vi "Core.vi"(8 "error in (no error)":errorcluster, 11 "Serial in":refnum<class "Serial.lvclass">) -> (0 "error out":errorcluster, 3 "Serial out":refnum<class "Serial.lvclass">)   [LabVIEW 2021, in "Serial.lvclass"]
uses:
  Serial.lvclass
  D:/my_projects/projects/Algorithms/Labview/21/Master CR/Master CR.lvclass
  ctl/CR_Core_State.ctl
  Master CR.lvclass/Master CR.ctl
  Status/Run/Write Run.vi
  Status/write/Write write.vi
  Modbus_v121c/Data Model/Device Data Model.lvclass
  Serial.lvclass/Serial.ctl
  Master CR.lvclass
  D:/my_projects/projects/Algorithms/Labview/21/Master CR/Devices/Serial/Serial.lvclass
panel:
  out "MB_TCP_State":T1=enum."requests"
  in  "write enable":bool=TRUE
  in  "stop":bool
  out "stopped":bool
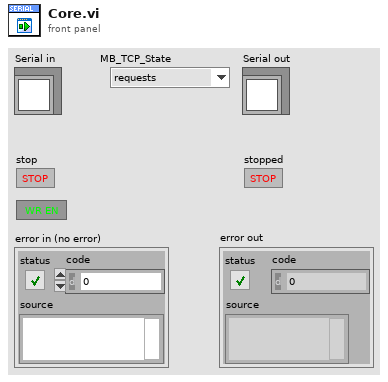
[diagram p1: front panel]
types:
  T1 = typedef "Master CR.lvclass/CR_Core_State.ctl" = enum8{"initialization", "redefine", "standby", "ping", "connect", "wait to reconnect", "wait to reset timeout", "configure", "requests", "close connection", "stop"}
  T2 = typedef "Master CR.lvclass/MB timeouts.ctl" = cluster{"reconn_timeout":i32, "N attempt max":i32, "t_reset_TTL":i32, "period":i32}
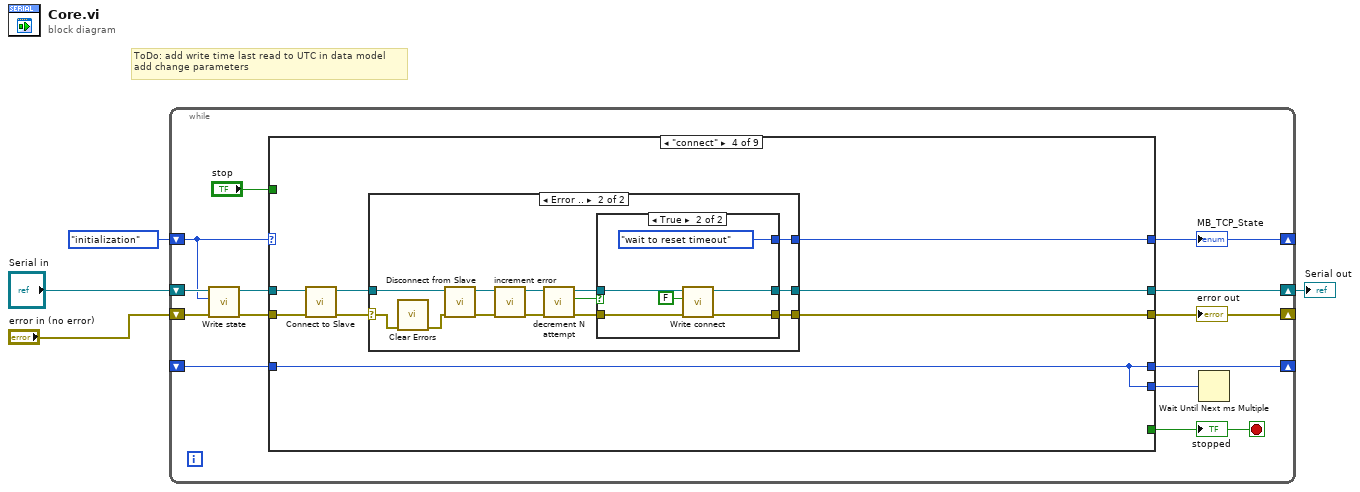
[diagram p0: block diagram]
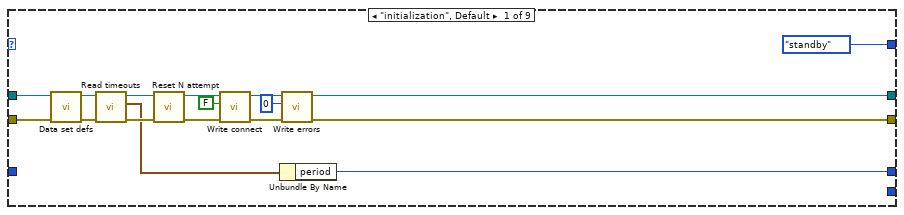
[diagram p2: hidden frame]
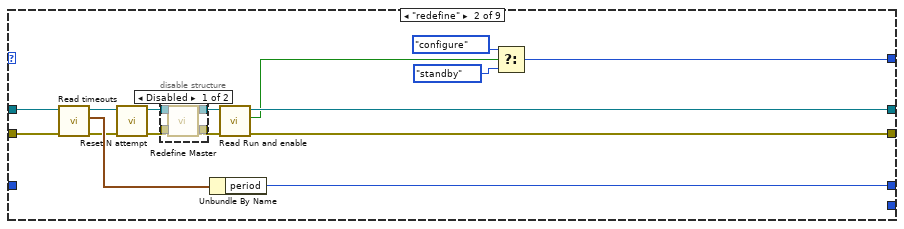
[diagram p3: hidden frame]
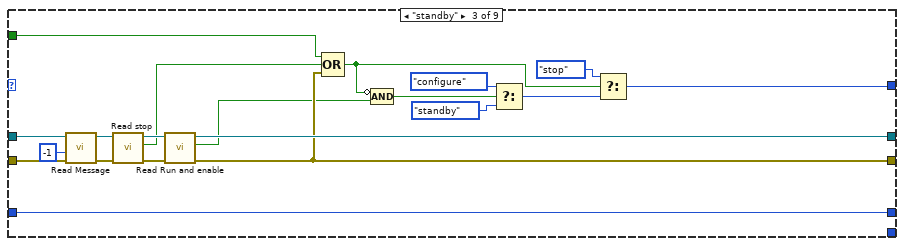
[diagram p5: hidden frame]
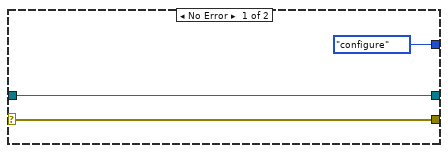
[diagram p6: hidden frame]
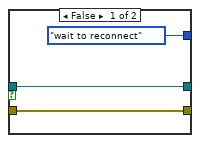
[diagram p7: hidden frame]
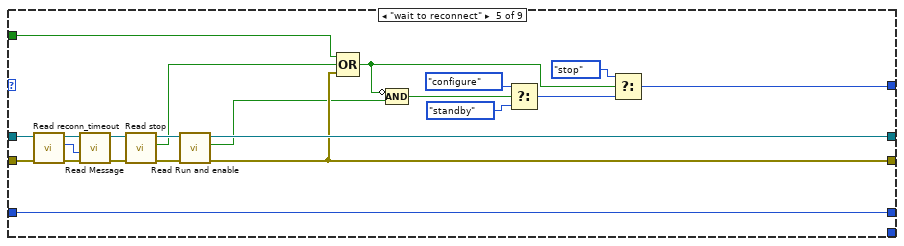
[diagram p8: hidden frame]
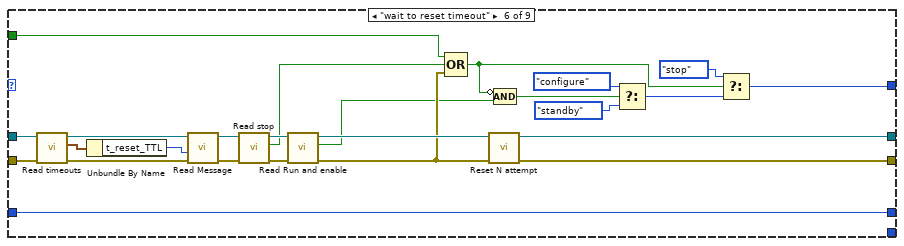
[diagram p9: hidden frame]
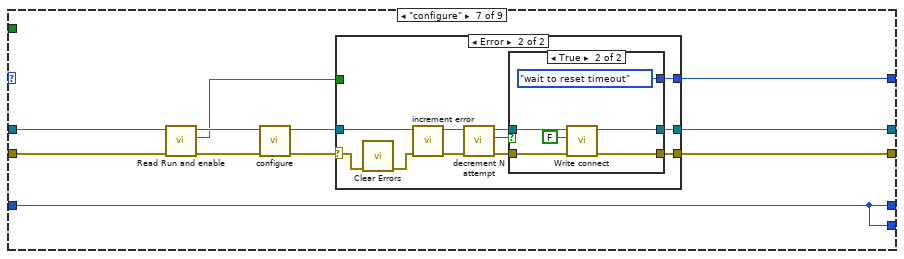
[diagram p10: hidden frame]
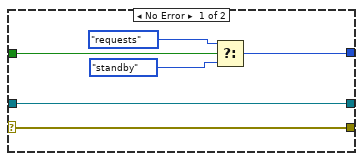
[diagram p11: hidden frame]
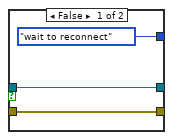
[diagram p12: hidden frame]
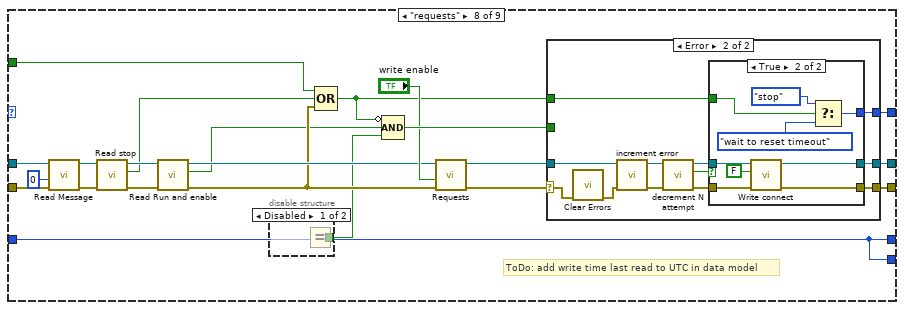
[diagram p13: hidden frame]
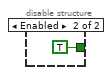
[diagram p14: hidden frame]
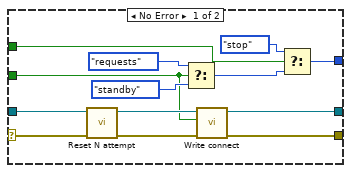
[diagram p15: hidden frame]
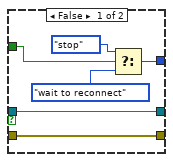
[diagram p16: hidden frame]
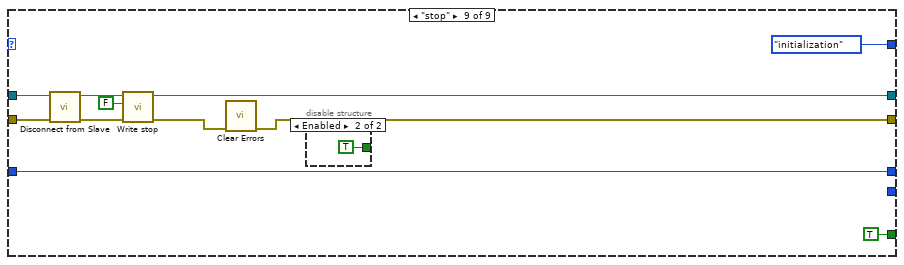
[diagram p17: hidden frame]
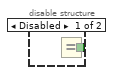
[diagram p18: hidden frame]
diagram:
  # "ToDo: add write time last read to UTC in data model\nadd change parameters"
  n1 = while {
    shift-right: [w10] -> w4
    shift-left: "Serial in" -> [w9]
    shift-right: [w11] -> _
    shift-left: "error in (no error)" -> [w7]
    shift-right: [w15] -> _
    shift-left: _ -> [w16]
    shift-right: [w12] -> _
    shift-left: CR_Core_State."initialization" ("state") -> [w5]
    stop <- w17 stop-if-true
    n2 = call "Write state.vi"("error in (no error)"=w7, "state"=w5, "Master CR in"=w9) -> ("error out"=w6:errorcluster, "Master CR out"=w8:refnum<class "Serial.lvclass">)  [unwired: 7 in]
    n3 = case shown="\"connect\"" w5 {
      tunnel: "stop" -> [_ _ w75 _ w119 w143 _ w205 _]
      tunnel: [_ _ _ _ _ _ _ _ TRUE] -> w17
      tunnel: w8 -> [w31 w47 w65 w80 w130 w155 w161 w207 w267]
      tunnel: [w20 w36 w67 w84 w117 w135 w167 w214 w260] -> w10
      tunnel: w6 -> [w32 w46 w64 w81 w129 w154 w160 w206 w266]
      tunnel: [CR_Core_State."standby" ("MB_TCP_State") w48 w68 w83 w118 w142 w166 w213 CR_Core_State."initialization" ("MB_TCP_State")] -> w12
      tunnel: [w18 w37 w66 w82 w116 w134 w165 w212 w265] -> w11
      tunnel: [w33 w44 w76 w77 w131 w156 w164 w210 w268] -> w15
      tunnel: w16 -> [_ _ w76 w77 w131 w156 w164 w210 w268]
      tunnel: [_ _ _ w77 _ _ w164 w210 _] -> w14
      frame "initialization", Default {
        n4 = call "Data set defs.vi"("error in (no error)"=w32, "Master CR in"=w31) -> ("error out"=w26:errorcluster, "Master CR out"=w29:refnum<class "Serial.lvclass">)  [unwired: 8 in]
        n5 = call "Read timeouts.vi"("error in (no error)"=w26, "Master CR in"=w29) -> ("error out"=w30:errorcluster, "MB timeouts"=w27:T2, "Master CR out"=w28:refnum<class "Serial.lvclass">)  [unwired: 7 in]
        n6 = call "Reset N attempt.vi"("error in (no error)"=w30, "Master CR in"=w28) -> ("error out"=w24:errorcluster, "Master CR out"=w25:refnum<class "Serial.lvclass">)  [unwired: 8 in]
        n7 = call "Write connect.vi"("error in (no error)"=w24, "connect"=FALSE, "Master CR in"=w25) -> ("error out"=w22:errorcluster, "Master CR out"=w21:refnum<class "Serial.lvclass">)  [unwired: 7 in]
        n8 = Unbundle By Name(w27) -> ("period"=w33:i32)
        n9 = call "Write errors.vi"("error in (no error)"=w22, "errors"=0, "Master CR in"=w21) -> ("error out"=w18:errorcluster, "Master CR out"=w20:refnum<class "Serial.lvclass">)  [unwired: 7 in]
      }
      frame "redefine" {
        n10 = call "Read timeouts.vi"("error in (no error)"=w46, "Master CR in"=w47) -> ("error out"=w43:errorcluster, "MB timeouts"=w45:T2, "Master CR out"=w42:refnum<class "Serial.lvclass">)  [unwired: 7 in]
        n11 = call "Reset N attempt.vi"("error in (no error)"=w43, "Master CR in"=w42) -> ("error out"=w40:errorcluster, "Master CR out"=w41:refnum<class "Serial.lvclass">)  [unwired: 8 in]
        n12 = disable-structure shown="Disabled" {
          disable-tunnel: w41 -> [w54 w56]
          disable-tunnel: w40 -> [w53 w55]
          disable-tunnel: [w52 w56] -> w39
          disable-tunnel: [w51 w55] -> w38
          frame Disabled {
            n13 = call "Redefine Master.vi"("error in (no error)"=w53, "Master CR in"=w54) -> ("error out"=w51:errorcluster, "Master CR out"=w52:refnum<class "Serial.lvclass">)  [unwired: 8 in]
          }
          frame Enabled {
          }
        }
        n14 = Unbundle By Name(w45) -> ("period"=w44:i32)
        n15 = call "Read Run and enable.vi"("error in (no error)"=w38, "Master CR in"=w39) -> ("error out"=w37:errorcluster, "Enable and Run"=w35:bool, "Master CR out"=w36:refnum<class "Serial.lvclass">)  [unwired: 7 in]
        n16 = Select(t=CR_Core_State."configure" ("MB_TCP_State"), s=w35, f=CR_Core_State."standby" ("MB_TCP_State")) -> (s? t:f=w48:T1)
      }
      frame "standby" {
        n17 = call "Read Message.vi"("error in (no error)"=w64, "timeout (0)"=-1, "Master CR in"=w65) -> ("error out"=w61:errorcluster, "Master CR out"=w62:refnum<class "Serial.lvclass">)  [unwired: 6 in, 1 out]
        n18 = call "Read stop.vi"("error in (no error)"=w61, "Master CR in"=w62) -> ("error out"=w60:errorcluster, "Stop"=w58:bool, "Master CR out"=w59:refnum<class "Serial.lvclass">)  [unwired: 7 in]
        n19 = call "Read Run and enable.vi"("error in (no error)"=w60, "Master CR in"=w59) -> ("error out"=w66:errorcluster, "Enable and Run"=w57:bool, "Master CR out"=w67:refnum<class "Serial.lvclass">)  [unwired: 7 in]
        n20 = Compound Arithmetic op=OR(w75, w58, w66) -> (w69:bool)
        n21 = Compound Arithmetic op=AND(invert w69, w57) -> (w70:bool)
        n22 = Select(t=CR_Core_State."configure" ("MB_TCP_State"), s=w70, f=CR_Core_State."standby" ("MB_TCP_State")) -> (s? t:f=w71:T1)
        n23 = Select(t=CR_Core_State."stop" ("MB_TCP_State"), s=w69, f=w71) -> (s? t:f=w68:T1)
      }
      frame "connect" {
        n24 = call-dynamic "Connect to Slave.vi"("error in (no error)"=w81, "network master in"=w80) -> ("error out"=w78:errorcluster, "network master out"=w79:refnum<class "Serial.lvclass">)  [unwired: 8 in]
        n25 = case shown="Error .." w78 {
          selector: w78 -> [w85 w92]
          tunnel: w79 -> [w86 w93]
          tunnel: [CR_Core_State."configure" ("MB_TCP_State") w98] -> w83
          tunnel: [w86 w97] -> w84
          tunnel: [w85 w96] -> w82
          frame No Error {
          }
          frame Error {
            n26 = call <vilib>:"Clear Errors.vi"("error in (no error)"=w92) -> ("error out"=w91:errorcluster)  [unwired: 5 in, 1 out]
            n27 = call-dynamic "Disconnect from Slave.vi"("error in (no error)"=w91, "network master in"=w93) -> ("error out"=w94:errorcluster, "network master out"=w95:refnum<class "Serial.lvclass">)  [unwired: 8 in]
            n28 = call "increment error.vi"("error in (no error)"=w94, "Master CR in"=w95) -> ("error out"=w90:errorcluster, "Master CR out"=w100:refnum<class "Serial.lvclass">)  [unwired: 7 in, 1 out]
            n29 = call "decrement N attempt.vi"("error in (no error)"=w90, "Master CR in"=w100) -> ("error out"=w88:errorcluster, "=0"=w99:bool, "Master CR out"=w89:refnum<class "Serial.lvclass">)  [unwired: 7 in]
            n30 = case shown="True" w99 {
              tunnel: [CR_Core_State."wait to reconnect" ("MB_TCP_State") CR_Core_State."wait to reset timeout" ("MB_TCP_State")] -> w98
              tunnel: w89 -> [w102 w105]
              tunnel: [w102 w108] -> w97
              tunnel: w88 -> [w101 w104]
              tunnel: [w101 w106] -> w96
              frame False {
              }
              frame True {
                n31 = call "Write connect.vi"("error in (no error)"=w104, "connect"=FALSE, "Master CR in"=w105) -> ("error out"=w106:errorcluster, "Master CR out"=w108:refnum<class "Serial.lvclass">)  [unwired: 7 in]
              }
            }
          }
        }
      }
      frame "wait to reconnect" {
        n32 = call "Read reconn_timeout.vi"("error in (no error)"=w129, "Master CR in"=w130) -> ("error out"=w120:errorcluster, "reconn_timeout"=w121:i32, "Master CR out"=w122:refnum<class "Serial.lvclass">)  [unwired: 7 in]
        n33 = call "Read Message.vi"("error in (no error)"=w120, "timeout (0)"=w121, "Master CR in"=w122) -> ("error out"=w114:errorcluster, "Master CR out"=w115:refnum<class "Serial.lvclass">)  [unwired: 6 in, 1 out]
        n34 = call "Read stop.vi"("error in (no error)"=w114, "Master CR in"=w115) -> ("error out"=w113:errorcluster, "Stop"=w111:bool, "Master CR out"=w112:refnum<class "Serial.lvclass">)  [unwired: 7 in]
        n35 = call "Read Run and enable.vi"("error in (no error)"=w113, "Master CR in"=w112) -> ("error out"=w116:errorcluster, "Enable and Run"=w110:bool, "Master CR out"=w117:refnum<class "Serial.lvclass">)  [unwired: 7 in]
        n36 = Compound Arithmetic op=OR(w119, w111, w116) -> (w123:bool)
        n37 = Compound Arithmetic op=AND(invert w123, w110) -> (w124:bool)
        n38 = Select(t=CR_Core_State."configure" ("MB_TCP_State"), s=w124, f=CR_Core_State."standby" ("MB_TCP_State")) -> (s? t:f=w125:T1)
        n39 = Select(t=CR_Core_State."stop" ("MB_TCP_State"), s=w123, f=w125) -> (s? t:f=w118:T1)
      }
      frame "wait to reset timeout" {
        n40 = call "Read timeouts.vi"("error in (no error)"=w154, "Master CR in"=w155) -> ("error out"=w146:errorcluster, "MB timeouts"=w153:T2, "Master CR out"=w145:refnum<class "Serial.lvclass">)  [unwired: 7 in]
        n41 = Unbundle By Name(w153) -> ("t_reset_TTL"=w144:i32)
        n42 = call "Read Message.vi"("error in (no error)"=w146, "timeout (0)"=w144, "Master CR in"=w145) -> ("error out"=w139:errorcluster, "Master CR out"=w141:refnum<class "Serial.lvclass">)  [unwired: 6 in, 1 out]
        n43 = call "Read stop.vi"("error in (no error)"=w139, "Master CR in"=w141) -> ("error out"=w138:errorcluster, "Stop"=w137:bool, "Master CR out"=w140:refnum<class "Serial.lvclass">)  [unwired: 7 in]
        n44 = call "Read Run and enable.vi"("error in (no error)"=w138, "Master CR in"=w140) -> ("error out"=w133:errorcluster, "Enable and Run"=w132:bool, "Master CR out"=w136:refnum<class "Serial.lvclass">)  [unwired: 7 in]
        n45 = Compound Arithmetic op=OR(w143, w137, w133) -> (w147:bool)
        n46 = call "Reset N attempt.vi"("error in (no error)"=w133, "Master CR in"=w136) -> ("error out"=w134:errorcluster, "Master CR out"=w135:refnum<class "Serial.lvclass">)  [unwired: 8 in]
        n47 = Compound Arithmetic op=AND(invert w147, w132) -> (w148:bool)
        n48 = Select(t=CR_Core_State."configure" ("MB_TCP_State"), s=w148, f=CR_Core_State."standby" ("MB_TCP_State")) -> (s? t:f=w149:T1)
        n49 = Select(t=CR_Core_State."stop" ("MB_TCP_State"), s=w147, f=w149) -> (s? t:f=w142:T1)
      }
      frame "configure" {
        n50 = call "Read Run and enable.vi"("error in (no error)"=w160, "Master CR in"=w161) -> ("error out"=w158:errorcluster, "Enable and Run"=w157:bool, "Master CR out"=w159:refnum<class "Serial.lvclass">)  [unwired: 7 in]
        n51 = call-dynamic "configure.vi"("error in (no error)"=w158, "Master CR in"=w159) -> ("error out"=w162:errorcluster, "Master CR out"=w163:refnum<class "Serial.lvclass">)  [unwired: 8 in]
        n52 = case shown="Error" w162 {
          selector: w162 -> [w169 w184]
          tunnel: [w173 w174] -> w166
          tunnel: [w169 w177] -> w165
          tunnel: w163 -> [w170 w176]
          tunnel: [w170 w178] -> w167
          tunnel: w157 -> [w168 _]
          frame No Error {
            n53 = Select(t=CR_Core_State."requests" ("MB_TCP_State"), s=w168, f=CR_Core_State."standby" ("MB_TCP_State")) -> (s? t:f=w173:T1)
          }
          frame Error {
            n54 = call <vilib>:"Clear Errors.vi"("error in (no error)"=w184) -> ("error out"=w175:errorcluster)  [unwired: 5 in, 1 out]
            n55 = call "increment error.vi"("error in (no error)"=w175, "Master CR in"=w176) -> ("error out"=w180:errorcluster, "Master CR out"=w179:refnum<class "Serial.lvclass">)  [unwired: 7 in, 1 out]
            n56 = call "decrement N attempt.vi"("error in (no error)"=w180, "Master CR in"=w179) -> ("error out"=w181:errorcluster, "=0"=w183:bool, "Master CR out"=w182:refnum<class "Serial.lvclass">)  [unwired: 7 in]
            n57 = case shown="True" w183 {
              tunnel: w182 -> [w187 w193]
              tunnel: [w187 w192] -> w178
              tunnel: w181 -> [w186 w191]
              tunnel: [w186 w189] -> w177
              tunnel: [CR_Core_State."wait to reconnect" ("MB_TCP_State") CR_Core_State."wait to reset timeout" ("MB_TCP_State")] -> w174
              frame False {
              }
              frame True {
                n58 = call "Write connect.vi"("error in (no error)"=w191, "connect"=FALSE, "Master CR in"=w193) -> ("error out"=w189:errorcluster, "Master CR out"=w192:refnum<class "Serial.lvclass">)  [unwired: 7 in]
              }
            }
          }
        }
      }
      frame "requests" {
        # "ToDo: add write time last read to UTC in data model"
        n59 = call "Read Message.vi"("error in (no error)"=w206, "timeout (0)"=0, "Master CR in"=w207) -> ("error out"=w200:errorcluster, "Master CR out"=w201:refnum<class "Serial.lvclass">)  [unwired: 6 in, 1 out]
        n60 = call "Read stop.vi"("error in (no error)"=w200, "Master CR in"=w201) -> ("error out"=w199:errorcluster, "Stop"=w197:bool, "Master CR out"=w198:refnum<class "Serial.lvclass">)  [unwired: 7 in]
        n61 = call "Read Run and enable.vi"("error in (no error)"=w199, "Master CR in"=w198) -> ("error out"=w203:errorcluster, "Enable and Run"=w194:bool, "Master CR out"=w204:refnum<class "Serial.lvclass">)  [unwired: 7 in]
        n62 = disable-structure shown="Disabled" {
          disable-tunnel: [w216 TRUE] -> w195
          frame Disabled {
            n63 = Equal?() -> (x = y?=w216:bool)  [unwired: 2 in]
          }
          frame Enabled {
          }
        }
        n64 = Compound Arithmetic op=OR(w205, w197, w203) -> (w196:bool)
        n65 = Compound Arithmetic op=AND(invert w196, w194, w195) -> (w215:bool)
        n66 = call-dynamic "Requests.vi"("error in (no error)"=w203, "write enable"="write enable", "Serial in"=w204) -> ("error out"=w208:errorcluster, "Serial out"=w211:refnum<class "Serial.lvclass">)  [unwired: 7 in]
        n67 = case shown="Error" w208 {
          selector: w208 -> [w227 w242]
          tunnel: [w220 w232] -> w213
          tunnel: w215 -> [w224 _]
          tunnel: [w222 w238] -> w212
          tunnel: w211 -> [w228 w235]
          tunnel: [w225 w239] -> w214
          tunnel: w196 -> [w218 w231]
          frame No Error {
            n68 = call "Reset N attempt.vi"("error in (no error)"=w227, "Master CR in"=w228) -> ("error out"=w223:errorcluster, "Master CR out"=w226:refnum<class "Serial.lvclass">)  [unwired: 8 in]
            n69 = Select(t=CR_Core_State."requests" ("MB_TCP_State"), s=w224, f=CR_Core_State."standby" ("MB_TCP_State")) -> (s? t:f=w219:T1)
            n70 = call "Write connect.vi"("error in (no error)"=w223, "connect"=w224, "Master CR in"=w226) -> ("error out"=w222:errorcluster, "Master CR out"=w225:refnum<class "Serial.lvclass">)  [unwired: 7 in]
            n71 = Select(t=CR_Core_State."stop" ("MB_TCP_State"), s=w218, f=w219) -> (s? t:f=w220:T1)
          }
          frame Error {
            n72 = call <vilib>:"Clear Errors.vi"("error in (no error)"=w242) -> ("error out"=w234:errorcluster)  [unwired: 5 in, 1 out]
            n73 = call "increment error.vi"("error in (no error)"=w234, "Master CR in"=w235) -> ("error out"=w236:errorcluster, "Master CR out"=w241:refnum<class "Serial.lvclass">)  [unwired: 7 in, 1 out]
            n74 = call "decrement N attempt.vi"("error in (no error)"=w236, "Master CR in"=w241) -> ("error out"=w237:errorcluster, "=0"=w233:bool, "Master CR out"=w240:refnum<class "Serial.lvclass">)  [unwired: 7 in]
            n75 = case shown="True" w233 {
              tunnel: w240 -> [w248 w257]
              tunnel: [w248 w256] -> w239
              tunnel: w237 -> [w247 w255]
              tunnel: [w247 w253] -> w238
              tunnel: [w245 w251] -> w232
              tunnel: w231 -> [w243 w249]
              frame False {
                n76 = Select(t=CR_Core_State."stop" ("MB_TCP_State"), s=w243, f=CR_Core_State."wait to reconnect" ("MB_TCP_State")) -> (s? t:f=w245:T1)
              }
              frame True {
                n77 = call "Write connect.vi"("error in (no error)"=w255, "connect"=FALSE, "Master CR in"=w257) -> ("error out"=w253:errorcluster, "Master CR out"=w256:refnum<class "Serial.lvclass">)  [unwired: 7 in]
                n78 = Select(t=CR_Core_State."stop" ("MB_TCP_State"), s=w249, f=CR_Core_State."wait to reset timeout" ("MB_TCP_State")) -> (s? t:f=w251:T1)
              }
            }
          }
        }
      }
      frame "stop" {
        n79 = call-dynamic "Disconnect from Slave.vi"("error in (no error)"=w266, "network master in"=w267) -> ("error out"=w259:errorcluster, "network master out"=w261:refnum<class "Serial.lvclass">)  [unwired: 8 in]
        n80 = call "Write stop.vi"("error in (no error)"=w259, "Stop"=FALSE, "Master CR in"=w261) -> ("error out"=w258:errorcluster, "Master CR out"=w260:refnum<class "Serial.lvclass">)  [unwired: 7 in]
        n81 = call <vilib>:"Clear Errors.vi"("error in (no error)"=w258) -> ("error out"=w265:errorcluster)  [unwired: 5 in, 1 out]
        n82 = disable-structure shown="Enabled" {
          disable-tunnel: [w269 TRUE] -> _
          frame Disabled {
            n83 = Equal?() -> (x = y?=w269:bool)  [unwired: 2 in]
          }
          frame Enabled {
          }
        }
      }
    }
    "stopped" <- w17
    "error out" <- w11
    "MB_TCP_State" <- w12
    n84 = Wait Until Next ms Multiple(millisecond multiple=w14) -> ()  [unwired: 1 out]
  }
  "Serial out" <- w4
